vi "Poly2path.vi"(11 "VertexArray":T1[](array[typedef])) -> (3 "Path":T2)   [LabVIEW 2014]
uses:
  TypeDefs/Point2DwSlope.ctl
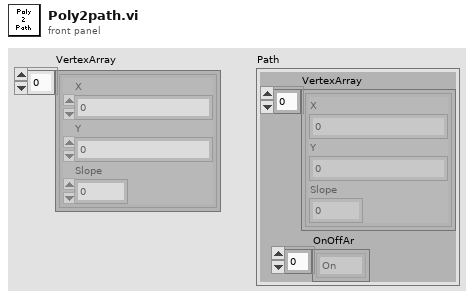
[diagram p1: front panel]
types:
  T1 = typedef "Point2DwSlope.ctl" = cluster{"X":sgl, "Y":sgl, "Slope":dbl}
  T2 = cluster{"VertexArray":T1[], "OnOffAr":enum16{"On", "Off"}[]}
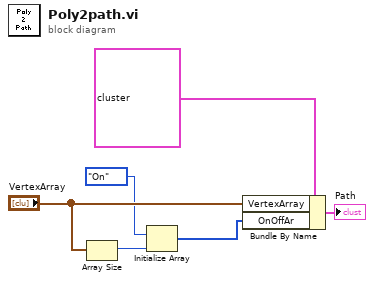
[diagram p0: block diagram]
diagram:
  n1 = Array Size(array="VertexArray") -> (size(s)=w4:i32)
  n2 = Initialize Array(enum16{"On", "Off"}."On", w4) -> (w3:enum16{"On", "Off"}[])
  n3 = Bundle By Name(cluster=T2 {"VertexArray"=[{"X"=-0.35355338, "Y"=-1.0606601, "Slope"=0.0}, {"X"=-0.35355338, "Y"=-1.0606601, "Slope"=0.0}, {"X"=-0.25355336, "Y"=-0.9606601, "Slope"=0.0}, {"X"=-0.4535534, "Y"=-0.9606601, "Slope"=0.0}, {"X"=-0.55355334, "Y"=-0.86066014, "Slope"=0.0}, {"X"=-0.1535534, "Y"=-0.86066014, "Slope"=0.0}, {"X"=-0.053553373, "Y"=-0.7606601, "Slope"=0.0}, {"X"=-0.65355337, "Y"=-0.7606601, "Slope"=0.0}, {"X"=-0.7535534, "Y"=-0.66066015, "Slope"=0.0}, {"X"=0.04644659, "Y"=-0.66066015, "Slope"=0.0}, {"X"=0.14644662, "Y"=-0.5606601, "Slope"=0.0}, {"X"=-0.8535534, "Y"=-0.5606601, "Slope"=0.0}, {"X"=-0.9535534, "Y"=-0.46066013, "Slope"=0.0}, {"X"=0.24644661, "Y"=-0.46066013, "Slope"=0.0}, {"X"=0.3464466, "Y"=-0.36066014, "Slope"=0.0}, {"X"=-1.0535533, "Y"=-0.36066014, "Slope"=0.0}, {"X"=-1.0606601, "Y"=-0.35355338, "Slope"=0.0}, {"X"=-1.0606601, "Y"=-0.35355338, "Slope"=0.0}, {"X"=-0.9677669, "Y"=-0.2606601, "Slope"=0.0}, {"X"=0.44644663, "Y"=-0.2606601, "Slope"=0.0}, {"X"=0.5464466, "Y"=-0.16066012, "Slope"=0.0}, {"X"=-0.86776686, "Y"=-0.16066012, "Slope"=0.0}, {"X"=-0.76776683, "Y"=-0.060660124, "Slope"=0.0}, {"X"=0.6464466, "Y"=-0.060660124, "Slope"=0.0}, {"X"=0.7464466, "Y"=0.039339878, "Slope"=0.0}, {"X"=-0.66776687, "Y"=0.039339878, "Slope"=0.0}, {"X"=-0.56776685, "Y"=0.13933988, "Slope"=0.0}, {"X"=0.84644663, "Y"=0.13933988, "Slope"=0.0}, {"X"=0.9464466, "Y"=0.23933987, "Slope"=0.0}, {"X"=-0.46776688, "Y"=0.23933987, "Slope"=0.0}, {"X"=-0.36776686, "Y"=0.33933988, "Slope"=0.0}, {"X"=1.0464466, "Y"=0.33933988, "Slope"=0.0}, {"X"=1.0606601, "Y"=0.35355338, "Slope"=0.0}, {"X"=1.0606601, "Y"=0.35355338, "Slope"=0.0}, {"X"=0.97487366, "Y"=0.43933988, "Slope"=0.0}, {"X"=-0.26776686, "Y"=0.43933988, "Slope"=0.0}, {"X"=-0.16776684, "Y"=0.5393399, "Slope"=0.0}, {"X"=0.87487364, "Y"=0.5393399, "Slope"=0.0}, {"X"=0.7748736, "Y"=0.63933986, "Slope"=0.0}, {"X"=-0.067766875, "Y"=0.63933986, "Slope"=0.0}, {"X"=0.03223315, "Y"=0.7393399, "Slope"=0.0}, {"X"=0.6748736, "Y"=0.7393399, "Slope"=0.0}, {"X"=0.5748737, "Y"=0.83933985, "Slope"=0.0}, {"X"=0.13223311, "Y"=0.83933985, "Slope"=0.0}, {"X"=0.23223314, "Y"=0.9393399, "Slope"=0.0}, {"X"=0.47487363, "Y"=0.9393399, "Slope"=0.0}, {"X"=0.3748736, "Y"=1.0393399, "Slope"=0.0}, {"X"=0.33223316, "Y"=1.0393399, "Slope"=0.0}], "OnOffAr"=[enum."On", enum."Off", enum."On", enum."Off", enum."On", enum."Off", enum."On", enum."Off", enum."On", enum."Off", enum."On", enum."Off", enum."On", enum."Off", enum."On", enum."Off", enum."On", enum."Off", enum."On", enum."Off", enum."On", enum."Off", enum."On", enum."Off", enum."On", enum."Off", enum."On", enum."Off", enum."On", enum."Off", enum."On", enum."Off", enum."On", enum."Off", enum."On", enum."Off", enum."On", enum."Off", enum."On", enum."Off", enum."On", enum."Off", enum."On", enum."Off", enum."On", enum."Off", enum."On", enum."Off"]} ("Path"), "VertexArray"="VertexArray", "OnOffAr"=w3) -> (→"Path":T2)
